vi "Clean Up Actor.vi"(8 "error in (no error)":errorcluster, 11 "WS Server in":refnum<class "WS Server.lvclass">) -> (0 "error out":errorcluster, 3 "WS Server out":refnum<class "WS Server.lvclass">)   [LabVIEW 2016, in "WebSocket Networking.lvlib" / "WS Server.lvclass"]
doc: "--\nCopyright © 2017 Composed SystemsI All rights reserved.\n\nAuthor: Jon McBee <jon.mcbee@composed.io>\n\nThis library is provided \"AS IS\" ,WITHOUT WARRANTIES OR\nCONDITIONS OF ANY KIND, either express or implied.\n\nComposed Systems -- composed.io\n\nStream 0.0.1.1\nJon McBee - Composed Systems\nCopyright (c) 2017, Composed Systems"
uses:
  <userlib>/Common Components/WebSocket Networking/WS Server/WS Server.lvclass
  C:/Program Files (x86)/National Instruments/LabVIEW 2016/user.lib/Composed Systems/Stream/Mediator/Classes/Mediated Actor/Mediated Actor.lvclass
  <userlib>/Common Components/WebSocket Networking/WS Server/WS Server.lvclass/WS Server.ctl
  <userlib>/Composed Systems/Stream/Mediator/Classes/Message Broker Interface/Message Broker Interface.lvclass
  <userlib>/Composed Systems/Stream/Mediator/Classes/Websocket Server Actor/Websocket Server/Websocket Server.lvclass
  <userlib>/Composed Systems/Stream/Mediator/Classes/Mediated Actor/Mediated Actor.lvclass
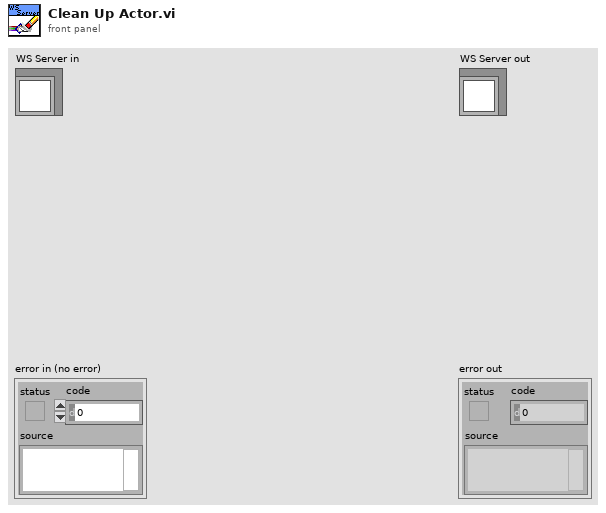
[diagram p1: front panel]
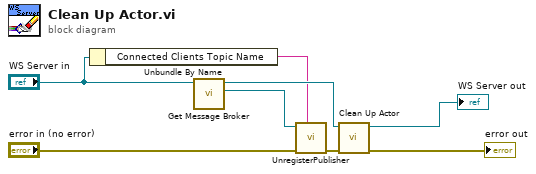
[diagram p0: block diagram]
diagram:
  n1 = Unbundle By Name("WS Server in") -> ("Connected Clients Topic Name"=w1:string)
  n2 = call <userlib>:"Get Message Broker.vi"("Mediated Actor in"="WS Server in") -> ("Message Broker"=w3:refnum<class "Message Broker Interface.lvclass">, "Mediated Actor out"=w5:refnum<class "WS Server.lvclass">)  [unwired: 9 in]
  n3 = call-dynamic "UnregisterPublisher.vi"("Topic Name"=w1, "error in (no error)"="error in (no error)", "Message Broker Interface in"=w3) -> ("error out"=w4:errorcluster)  [unwired: 7 in, 1 out]
  n4 = call-parent "Clean Up Actor.vi"("error in (no error)"=w4, "Mediated Asynchronous Actor in"=w5) -> ("error out"=→"error out":errorcluster, "Mediated Asynchronous Actor out"=→"WS Server out":refnum<class "WS Server.lvclass">)  [unwired: 8 in]
